vi "Subtractor3.vi"() -> (8 "Subtractor3":refnum<class "Subtractor3.lvclass">)   [LabVIEW 2017, in "Subtractor3.lvclass"]
uses:
  Subtractor3.lvclass
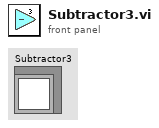
[diagram p1: front panel]
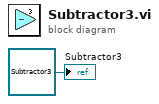
[diagram p0: block diagram]
diagram:
  "Subtractor3" <- refnum<class "Subtractor3.lvclass"> refnum ("Subtractor3.lvclass")
